vi "Write.vi"(11 "Scaled MV":dbl(slide) scale=0.0..2000.0) -> ()   [LabVIEW 2018]
uses:
  <vilib>/DAQmx/write.llb/DAQmx Write (Analog DBL 1Chan 1Samp).vi
  <vilib>/DAQmx/create/channels.llb/DAQmx Create Channel (AI-Voltage-Basic).vi
  <vilib>/DAQmx/miscellaneous.llb/DAQmx Fill In Error Info.vi
panel:
  in  "stop":bool
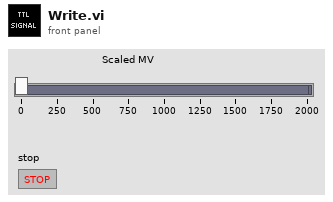
[diagram p1: front panel]
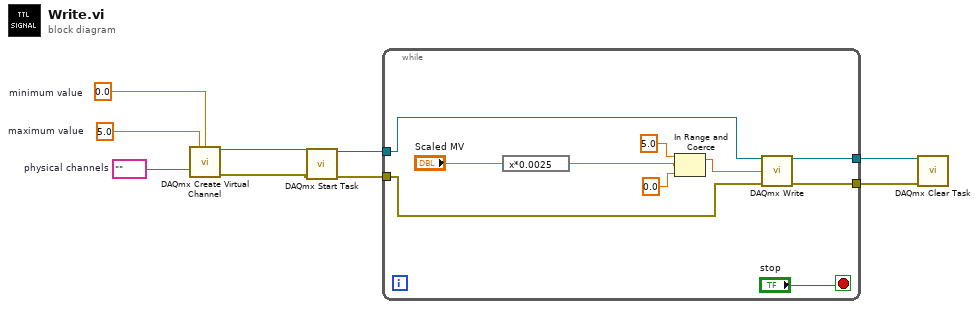
[diagram p0: block diagram]
diagram:
  w3 = tag ""  # physical channels
  w4 = 0.0  # minimum value
  w5 = 5.0  # maximum value
  n1 = call-poly <vilib>:"DAQmx Create Virtual Channel.vi"("maximum value"=w5, "minimum value"=w4, "physical channels"=w3) -> ("task out"=w7:refnum<k21>, "error out"=w6:errorcluster)  [unwired: 11 in]
  n2 = call <vilib>:"DAQmx Start Task.vi"("task/channels in"=w7, "error in"=w6) -> ("task out"=w2:refnum<k21>, "error out"=w1:errorcluster)  [unwired: 12 in]
  n3 = while {
    tunnel: [w17] -> w9
    tunnel: [w16] -> w8
    tunnel: w2 -> [w11]
    tunnel: w1 -> [w10]
    stop <- "stop" stop-if-true
    n4 = expression code="x*0.0025"("Scaled MV") -> (w14:dbl)
    n5 = In Range and Coerce(upper limit=5.0, x=w14, lower limit=0.0) -> (coerced(x)=w15:dbl)  [unwired: 1 out]
    n6 = call-poly <vilib>:"DAQmx Write.vi"("task/channels in"=w11, "data"=w15, "error in"=w10) -> ("task out"=w17:refnum<k21>, "error out"=w16:errorcluster)  [unwired: 10 in, 1 out]
  }
  n7 = call <vilib>:"DAQmx Clear Task.vi"("task in"=w9, "error in"=w8) -> ()  [unwired: 13 in, 1 out]
